vi "Read Name core.vi"(11 "Open VIPM Step in":refnum<class "Open VIPM Step.lvclass">) -> (2 "Name":string)   [LabVIEW 2019, in "VIPM.lvlib" / "Open VIPM Step.lvclass"]
doc: "Gets the name for the build step\n\nCopyright: MGI 2016\nAuthor: Derek Trepanier"
uses:
  Open VIPM Step.lvclass
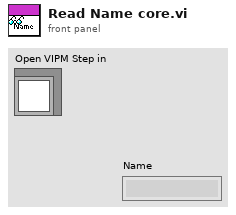
[diagram p1: front panel]
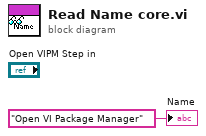
[diagram p0: block diagram]
diagram:
  "Name" <- "Open VI Package Manager" ("Name")
